vi "OTD Annual Report Example 2014yr.vi"() -> ()   [LabVIEW 2014]
uses:
  <vilib>/addons/database/Connection.llb/DB Tools Open Connec (Path).vi
  <userlib>/_OpenG.lib/array/array.llb/Search 1D Array (Boolean)__ogtk.vi
  <vilib>/addons/database/NI_Database_API.lvlib
panel:
  out "x-y 2":dbl
  out "x-y":dbl
  out "sum 2":i32
  out "Array 2":i32[](array[numeric])
  out "Annual Report 2":cluster{dbl[], dbl[]}[](graph)
  out "size(s)":i32
  out "Table 2":string[][](table)=[["34", "74", "23", "35", "23", "26", "74", "74", "21", "39", "61", "83"], ["73", "24", "75", "87", "42", "34", "35", "76", "52", "43", "43", "3"], ["36", "25", "12", "34", "24", "74", "73", "54", "88", "64", "90", "62"]]
  out "Array":i32[](array[numeric])
  out "data":string[][](table)
  # "Jan"
  # "Feb"
  # "Mar"
  # "April"
  # "May"
  # "June"
  # "July"
  # "Aug"
  # "Sept"
  # "Oct"
  # "Nov"
  # "Dec"
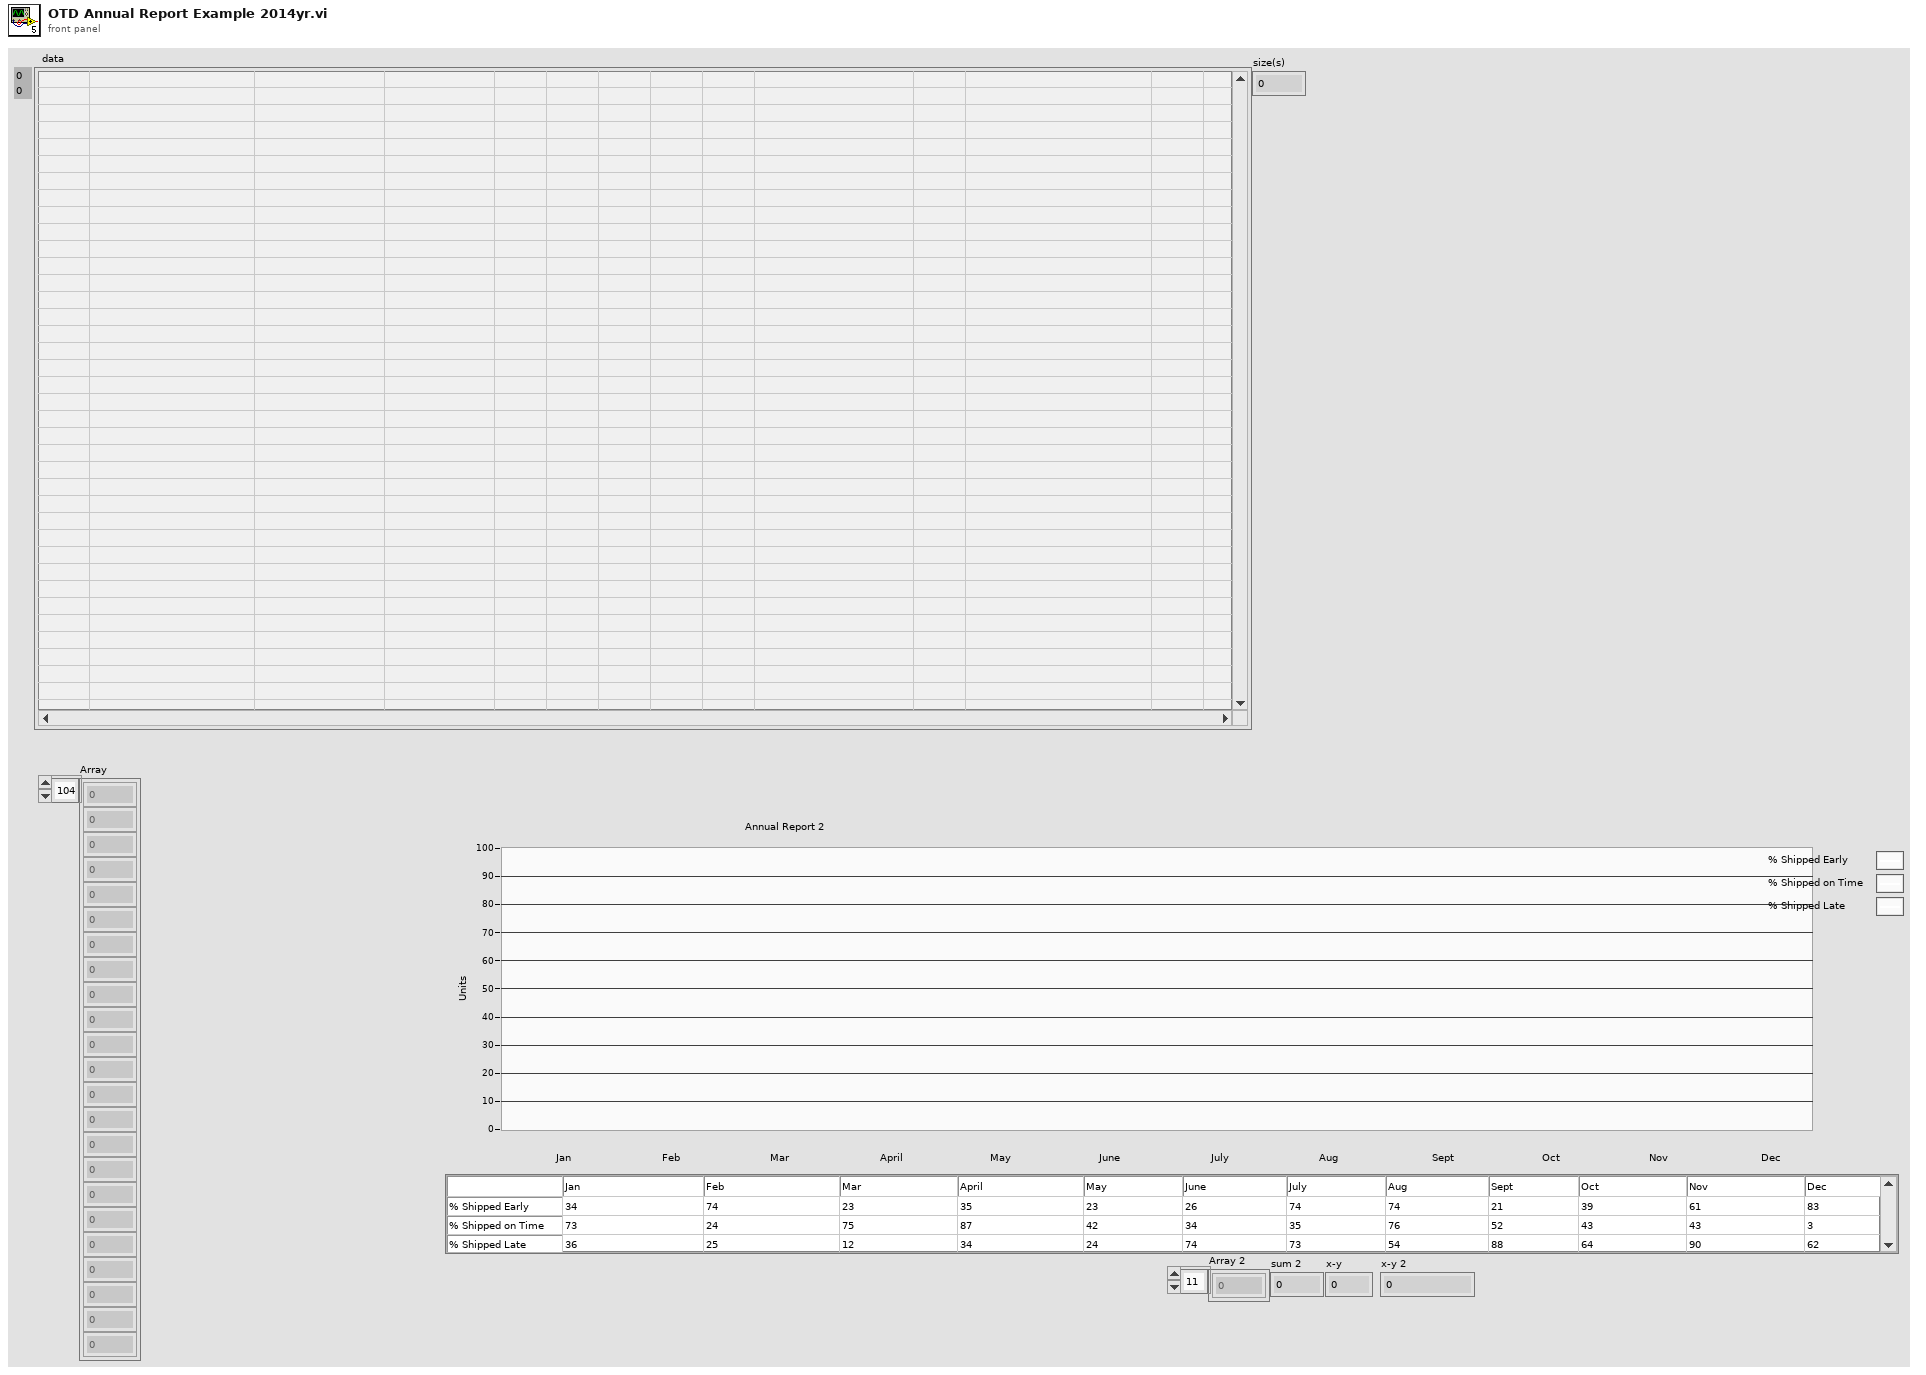
[diagram p1: front panel]
types:
  T1 = cluster{"Begin Date":string, "End Date":string}[]
  T2 = typedef "NI_Database_API.lvlib/Conn ObjectReference.ctl" = refnum<k1>
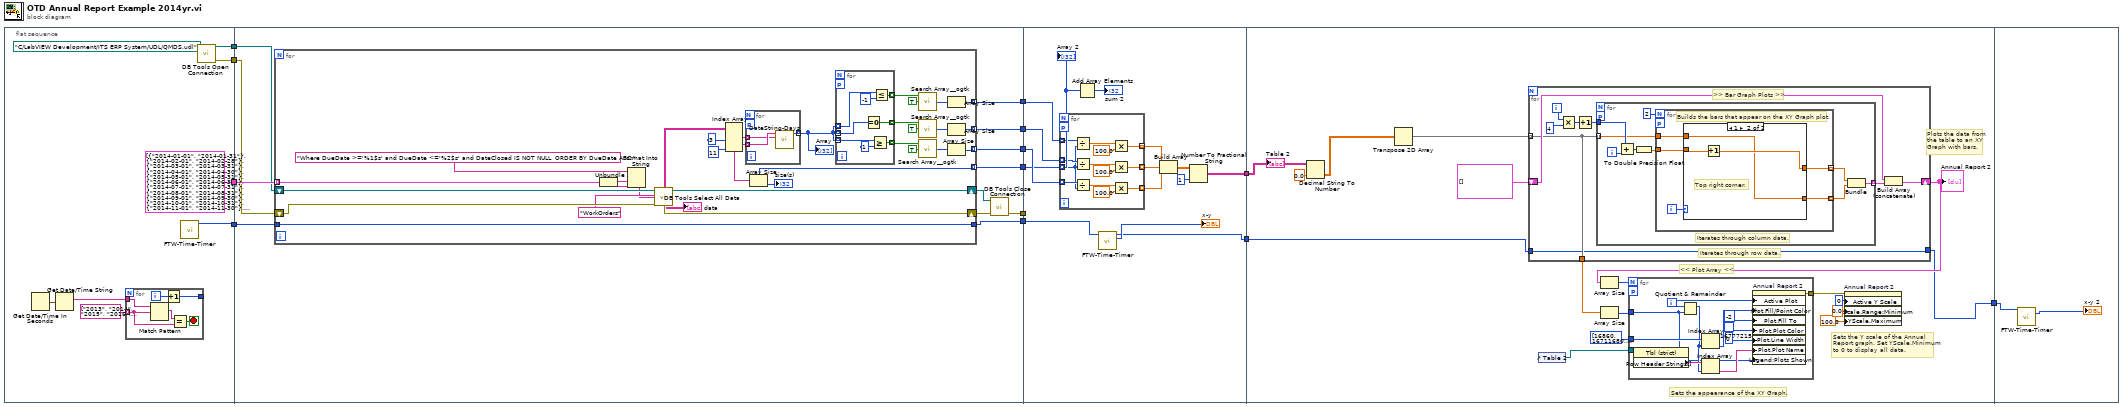
[diagram p0: block diagram]
diagram:
  n1 = flat-sequence {
    tunnel: [w20] -> w13
    tunnel: [w19] -> w12
    tunnel: [T1 [{"Begin Date"="2014-01-01", "End Date"="2014-01-31"}, {"Begin Date"="2014-02-01", "End Date"="2014-02-28"}, {"Begin Date"="2014-03-01", "End Date"="2014-03-31"}, {"Begin Date"="2014-04-01", "End Date"="2014-04-30"}, {"Begin Date"="2014-05-01", "End Date"="2014-05-31"}, {"Begin Date"="2014-06-01", "End Date"="2014-06-30"}, {"Begin Date"="2014-07-01", "End Date"="2014-07-31"}, {"Begin Date"="2014-08-01", "End Date"="2014-08-31"}, {"Begin Date"="2014-09-01", "End Date"="2014-09-30"}, {"Begin Date"="2014-10-01", "End Date"="2014-10-31"}, {"Begin Date"="2014-11-01", "End Date"="2014-11-30"}, {"Begin Date"="2014-12-01", "End Date"="2014-12-31"}]] -> w11
    tunnel: [w17] -> w10
    tunnel: w13 -> [w29]
    tunnel: w12 -> [w28]
    tunnel: w11 -> [w39]
    tunnel: w10 -> [w36]
    tunnel: [w35] -> w9
    tunnel: [w34] -> w8
    tunnel: [w33] -> w7
    tunnel: [w32] -> w6
    tunnel: [w31] -> w5
    tunnel: [w30] -> w4
    tunnel: w9 -> [_]
    tunnel: w8 -> [w83]
    tunnel: w7 -> [w85]
    tunnel: w6 -> [w88]
    tunnel: w5 -> [w87]
    tunnel: w4 -> [w86]
    tunnel: [w84] -> w3
    tunnel: [w81] -> w2
    tunnel: w3 -> [w110]
    tunnel: w2 -> [w109]
    tunnel: [w108] -> w1
    tunnel: w1 -> [w166]
    frame #0 {
      n2 = Get Date/Time In Seconds() -> (seconds since 1Jan1904=w16:timestamp)
      n3 = Get Date/Time String(seconds (now)=w16) -> (date string=w15:string)  [unwired: 2 in, 1 out]
      n4 = for {
        tunnel: w15 -> [w27]
        tunnel: string[] ["2013", "2014", "2015", "2016", "2017", "2018"] -> [w23] mode=indexing
        tunnel: [w25] -> _
        i -> [w26]
        stop <- w22 stop-if-true
        n5 = Match Pattern(string=w27, regular expression=w23) -> (match substring=w24:string)  [unwired: 1 in, 3 out]
        n6 = Increment(x=w26) -> (x+1=w25:i32)
        n7 = Equal?(x=w24, y=w23) -> (x = y?=w22:bool)
      }
      n8 = call "FTW-Time-Timer.vi"() -> ("Current Tick Count"=w17:u32)  [unwired: 13 in, 2 out]
      n9 = call-poly <vilib>:"DB Tools Open Connection.vi"("connection information"=path "C:/LabVIEW Development/ITS ERP System/UDL/QMDS.udl" ("Database (mdb)  File Path")) -> ("error out"=w19:errorcluster, "connection reference"=w20:T2)  [unwired: 7 in]
    }
    frame #1 {
      n10 = for {
        tunnel: [w59] -> w33 mode=indexing
        shift-right: [w66] -> w38
        shift-left: w29 -> [w69]
        shift-right: [w65] -> w37
        shift-left: w28 -> [w68]
        tunnel: [w54] -> w32 mode=indexing
        tunnel: [w47] -> w30 mode=indexing
        tunnel: [w46] -> w31 mode=indexing
        tunnel: w39 -> [w45] mode=indexing
        tunnel: [w40] -> w34
        tunnel: w36 -> [w40]
        n11 = Unbundle(w45) -> ("Begin Date"=w44:string, "End Date"=w43:string)
        n12 = Format Into String(format string="Where DueDate >='%1$s' and DueDate <='%2$s' and DateClosed IS NOT NULL  ORDER BY DueDate ASC;" ("optional clause"), w44, w43) -> (resulting string=w42:string)  [unwired: 2 in, 1 out]
        n13 = call <vilib>:"DB Tools Select All Data.vi"("optional clause"=w42, "error in (no error)"=w68, "table"="WorkOrders" ("Table"), "connection reference"=w69) -> ("error out"=w65:errorcluster, "data"=w64:string[][], "connection reference out"=w66:T2)  [unwired: 2 in]
        "data" <- w64
        n14 = Index Array(array=w64, index (col) #1=3 ("disabled index (col)"), index (col) #2=11 ("index (col)")) -> (element #1=w61:string[], element #2=w60:string[])  [unwired: 2 in]
        n15 = for {
          tunnel: w61 -> [w78] mode=indexing
          tunnel: w60 -> [w79] mode=indexing
          tunnel: [w80] -> w58 mode=indexing
          workers-P: _ -> [_]
          n16 = call "DateString-Days.vi"("First date"=w78, "Second date"=w79) -> ("Elapsed days"=w80:i32)  [unwired: 8 in, 1 out]
        }
        "Array" <- w58
        n17 = Array Size(array=w60) -> (size(s)=w59:i32)
        "size(s)" <- w59
        n18 = for {
          tunnel: w58 -> [w75] mode=indexing
          tunnel: [w76] -> w55 mode=indexing
          tunnel: w58 -> [w74] mode=indexing
          tunnel: w58 -> [w72] mode=indexing
          tunnel: [w71] -> w51 mode=indexing
          tunnel: [w70] -> w48 mode=indexing
          workers-P: _ -> [_]
          n19 = Equal To 0?(x=w74) -> (x = 0?=w71:bool)
          n20 = Greater Or Equal?(x=w72, y=1) -> (x >= y?=w70:bool)
          n21 = Less Or Equal?(x=w75, y=-1) -> (x <= y?=w76:bool)
        }
        n22 = call-poly <userlib>:"Search Array__ogtk.vi"("Array"=w55, "Element Data"=TRUE) -> ("Indices of Elements"=w57:i32[])  [unwired: 7 in]
        n23 = call-poly <userlib>:"Search Array__ogtk.vi"("Array"=w51, "Element Data"=TRUE) -> ("Indices of Elements"=w52:i32[])  [unwired: 7 in]
        n24 = call-poly <userlib>:"Search Array__ogtk.vi"("Array"=w48, "Element Data"=TRUE) -> ("Indices of Elements"=w50:i32[])  [unwired: 7 in]
        n25 = Array Size(array=w57) -> (size(s)=w54:i32)
        n26 = Array Size(array=w52) -> (size(s)=w46:i32)
        n27 = Array Size(array=w50) -> (size(s)=w47:i32)
      }
      n28 = call <vilib>:"DB Tools Close Connection.vi"("error in (no error)"=w37, "connection reference"=w38) -> ("error out"=w35:errorcluster)  [unwired: 5 in]
    }
    frame #2 {
      n29 = for {
        tunnel: w88 -> [w107] mode=indexing
        tunnel: w85 -> [w97] mode=indexing
        tunnel: [w104] -> w89 mode=indexing
        tunnel: w87 -> [w99] mode=indexing
        tunnel: w86 -> [w98] mode=indexing
        tunnel: [w96] -> w92 mode=indexing
        tunnel: [w95] -> w93 mode=indexing
        workers-P: _ -> [_]
        n30 = Divide(x=w107, y=w97) -> (x/y=w106:dbl)
        n31 = Divide(x=w99, y=w97) -> (x/y=w102:dbl)
        n32 = Divide(x=w98, y=w97) -> (x/y=w101:dbl)
        n33 = Multiply(x=w106, y=100.0) -> (x*y=w104:dbl)
        n34 = Multiply(x=w102, y=100.0) -> (x*y=w96:dbl)
        n35 = Multiply(x=w101, y=100.0) -> (x*y=w95:dbl)
      }
      n36 = Add Array Elements(numeric array=w85) -> (sum=→"sum 2":i32)
      n37 = call "FTW-Time-Timer.vi"("Initial Tick Count"=w83) -> ("Current Tick Count"=w81:u32, "Elapsed Time"=→"x-y":u32)  [unwired: 12 in, 1 out]
      n38 = Build Array(w89, w92, w93) -> (w90:dbl[][])
      n39 = Number To Fractional String(number=w90, precision (6)=i16 1) -> (F-format string=w84:string[][])  [unwired: 2 in]
      "Array 2" <- w85
    }
    frame #3 {
      # "Plots the data from the table to an XY Graph with bars."
      # "Sets the appearance of the XY Graph."
      # "Sets the Y scale of the Annual Report graph. Set YScale.Minimum to 0 to display all data."
      # "<< Plot Array <<"
      n40 = Decimal String To Number(string=w110, default (0L)=0.0) -> (number=w122:dbl[][])  [unwired: 2 out]
      n41 = Transpose 2D Array(2D array=w122) -> (transposed array=w121:dbl[][])
      n42 = for {
        tunnel: w121 -> [w138] mode=indexing
        shift-right: [w142] -> w119
        shift-left: cluster{dbl[], dbl[]}[] [] -> [w141]
        tunnel: [w138] -> w117
        tunnel: [w137] -> w108
        tunnel: w109 -> [w137]
        i -> [w145]
        # "Iterates through row data."
        # ">> Bar Graph Plots >>"
        n43 = Multiply(x=w145, y=4) -> (x*y=w140:i32)
        n44 = Increment(x=w140) -> (x+1=w139:i32)
        n45 = for {
          tunnel: w138 -> [w147] mode=indexing
          tunnel: w139 -> [w154]
          tunnel: [w149] -> w143 mode=indexing
          workers-P: _ -> [_]
          i -> [w148]
          # "Iterates through column data."
          n46 = Add(x=w154, y=w148) -> (x+y=w153:i32)
          n47 = To Double Precision Float(number=w153) -> (double precision float=w152:dbl)
          n48 = for {
            N: 2 -> [_]
            tunnel: w147 -> [w158]
            tunnel: [w157] -> w150 mode=indexing
            tunnel: w152 -> [w156]
            tunnel: [w155] -> w151 mode=indexing
            workers-P: _ -> [_]
            i -> [w159]
            # "Builds the bars that appear on the XY Graph plot."
            n49 = case shown="1" w159 {
              tunnel: w158 -> [w161 w162]
              tunnel: [w161 w162] -> w157
              tunnel: w156 -> [w160 w164]
              tunnel: [w160 w163] -> w155
              frame 0, Default {
                # "Top left corner."
              }
              frame 1 {
                # "Top right corner."
                n50 = Increment(x=w164) -> (x+1=w163:dbl)
              }
            }
          }
          n51 = Bundle(w151, w150) -> (w149:cluster{dbl[], dbl[]})  [unwired: 1 out]
        }
        n52 = Build Array (concatenate) "Build Array"(w141, w143) -> (w142:cluster{dbl[], dbl[]}[])
      }
      "Annual Report 2" <- w119
      n53 = control-ref of="Table 2"() -> (w124:refnum<vi>)
      n54 = Array Size(array=w119) -> (size(s)=w118:i32)
      n55 = Array Size(array=w117) -> (size(s)=w116:i32)
      n56 = for {
        N: w118 -> [_]
        tunnel: w116 -> [w127]
        tunnel: u32[] [16860, 16711680, 1175296, 16773632, 15679744, 16711925, 2818015, 4325415] -> [w132]
        tunnel: [w126] -> w114
        tunnel: w124 -> [w125]
        workers-P: _ -> [_]
        i -> [w136]
        n57 = property on="Property Node" class="Tbl (strict)"(reference=w125) -> ("Row Header Strings[]"=w130:string[])  [unwired: 1 in, 2 out]
        n58 = Quotient & Remainder(x=w136, y=w127) -> (x-y*floor(x/y)=w129:i32)  [unwired: 1 out]
        n59 = Index Array(array=w132, index=w129) -> (element=w135:u32)
        n60 = Index Array(array=w130, index=w129) -> (element=w128:string)
        n61 = property on="Annual Report 2" class="XYGraph (strict)"("Active Plot"=w136, "Plot.Fill/Point Color"=w135, "Plot.Fill To"=i16 -2, "Plot.Plot Color"=u32 16777215, "Plot.Line Width"=u8 0, "Plot.Plot Name"=w128, "Legend:Plots Shown"=w127) -> (error out=w126:errorcluster)  [unwired: 2 in, 1 out]
      }
      n62 = property on="Annual Report 2" class="XYGraph (strict)"(error in=w114, "Active Y Scale"=0 ("Active X Scale"), "Y Scale.Range:Minimum"=0.0 ("X Scale.Range:Maximum"), "YScale.Maximum"=100.0 ("Y Scale.Range:Maximum")) -> ()  [unwired: 1 in, 2 out]
      "Table 2" <- w110
    }
    frame #4 {
      n63 = call "FTW-Time-Timer.vi"("Initial Tick Count"=w166) -> ("Elapsed Time"=→"x-y 2":u32)  [unwired: 12 in, 2 out]
    }
  }
